vi "IMU-UART-String-to-Euler.vi"(0 "IMU Data":string) -> (1 "xAccel":dbl, 2 "yAccel":dbl, 3 "zAccel":dbl, 4 "roll":dbl, 6 "pitch":dbl, 8 "yaw":dbl(graph))   [LabVIEW 2017]
panel:
  out "*(type *) &x":u8[](array[numeric])
  out "Output String":string
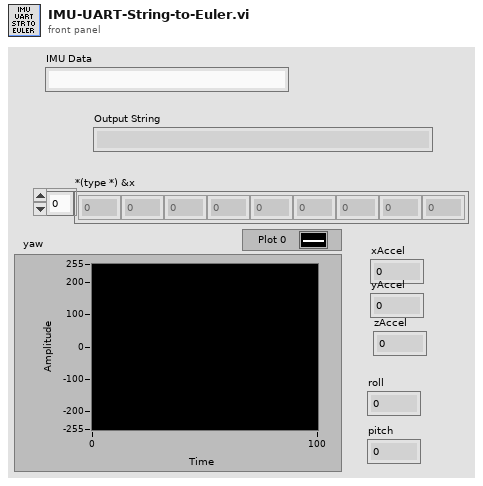
[diagram p1: front panel]
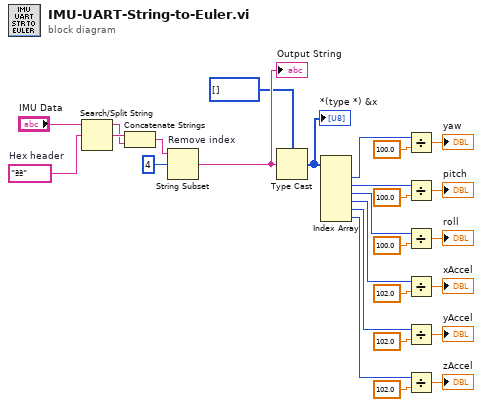
[diagram p0: block diagram]
diagram:
  w19 = "ªª"  # Hex header
  n1 = Search/Split String(string="IMU Data", search string/char (-)=w19) -> (substring before match=w20:string, match + rest of string=w21:string)  [unwired: 1 in, 1 out]
  n2 = Concatenate Strings(w21, w20) -> (w23:string)
  n3 = String Subset "Remove index"(string=w23, offset (0)=4) -> (substring=w25:string)  [unwired: 1 in]
  "Output String" <- w25
  n4 = Type Cast(type=i16[] [], x=w25) -> (*(type *) &x=w26:i16[])
  "*(type *) &x" <- w26
  n5 = Index Array(array=w26) -> (element #1=w17:i16, element #2=w13:i16, element #3=w12:i16, element #4=w3:i16, element #5=w2:i16, element #6=w1:i16)  [unwired: 6 in]
  n6 = Divide(x=w17, y=100.0) -> (x/y=→"yaw":dbl)
  n7 = Divide(x=w13, y=100.0) -> (x/y=→"pitch":dbl)
  n8 = Divide(x=w12, y=100.0) -> (x/y=→"roll":dbl)
  n9 = Divide(x=w3, y=102.0) -> (x/y=→"xAccel":dbl)
  n10 = Divide(x=w2, y=102.0) -> (x/y=→"yAccel":dbl)
  n11 = Divide(x=w1, y=102.0) -> (x/y=→"zAccel":dbl)
